vi "Global 1.vi"() -> ()   [LabVIEW 2019]
panel:
  out "Boolean 2":bool
  in  "Boolean":bool
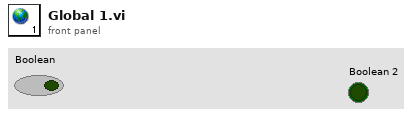
[diagram p1: front panel]
diagram:
